vi "_Server BlockUpdate.vi"(4 "error in":errorcluster, 5 "Simulator":bool, 6 "Lens":T1[](array[typedef]), 7 "Running":bool) -> (0 "error out":errorcluster)   [LabVIEW 2015]
uses:
  Type/_XML Lens.ctl
  Type/_RT Active Ch.ctl
  Type/_RT Parameter.ctl
  Type/_RT Expt.ctl
  Type/_Run Mode.ctl
  Type/_RT Mass Range.ctl
  Type/_RT Res Type.ctl
  Type/_RT Command.ctl
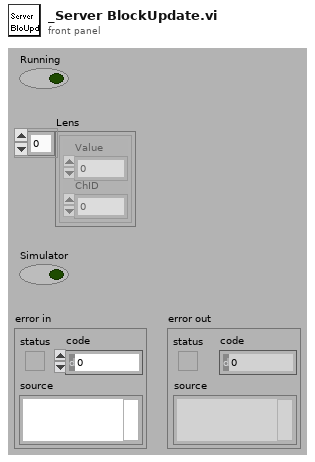
[diagram p1: front panel]
types:
  T1 = typedef "_XML Lens.ctl" = cluster{"Value":dbl, "ChID":u8}
  T2 = typedef "_RT Command.ctl" = enum16{"xml Start Run", "xml Start Actual Run", "xml Stop Run", "xml Runtime Update", "xml Get Status", "xml Get Table", "xml Set Table", "xml Get Configuration", "xml System Status", "xml Set LC Input Logic", "xml Get Data", "xml Get Info", "Start", "StartActualRun", "Stop", "Runtime Update", "Get Data", "Get Info", "Get Status", "Get Param", "Get Config", "Get Table", "Read ADC", "Set Oscillator", "Update Config", "Update Table", "Set All Pol", "Set Pol and DC", "Set Max Mass", "Toggle RP", "Toggle EL", "Set PIC", "Initialize Turbo", "Send Turbo Comm", "Close Turbo", "P1", "P2", "P3", "Send Serial", "Set LC Out", "Get LC In", "Read VAC", "Test Table", "Toggle Power", "Get Startup", "Set Startup", "Get ADC Table", "Set ADC Table", "Get Brief Status", "Get Detail Status", "Auxiliary Update", "Set CC Logics", "Set CC Input Logics", "Ignore Error", "invalid"}
  T3 = typedef "_RT Active Ch.ctl" = cluster{"Start":i32, "Step":i32, "ChID":i32}
  T4 = typedef "_RT Configuration 2.ctl" = cluster{"Name":string, "Ch#":u8, "Min":dbl, "Max":dbl, "Def+":dbl, "Def-":dbl, "Offset":dbl, "Slope":dbl, "Type":u8, "Description":string, "SettleT":dbl}
  T5 = typedef "_RT Expt.ctl" = cluster{"StartT(mS)":i32, "#Cycles":i32, "Scan Type":T6, "PauseT(uS)":i32, "Polarity":u8, "DelayT(mS)":i32, "Active Ch":T3[], "Mass Range":T7[]}
  T6 = typedef "_Run Mode.ctl" = enum16{"MRM (Q1/Q2)", "Q1 Scan", "Q1 SRM", "Q2 Scan", "Q2 SRM", "Product Scan", "Precursor Scan", "Neutral Loss", "Neutral Gain"}
  T7 = typedef "_RT Mass Range.ctl" = cluster{"Steps":i32, "Dwell(uS)":i32, "Resolution Type":T8, "Ramping Ch":T3[]}
  T8 = typedef "_RT Res Type.ctl" = u16
  T9 = typedef "_RT Parameter.ctl" = cluster{"RunMode":i32, "Initial Ch":T3[], "Sync":u8, "Expt":T5[], "EqTime(mS)":i32}
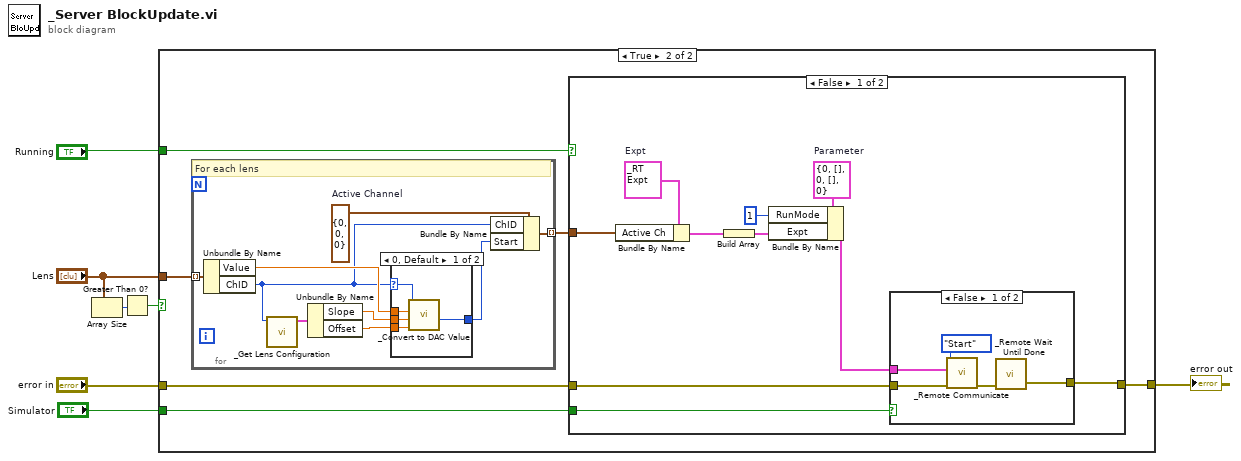
[diagram p0: block diagram]
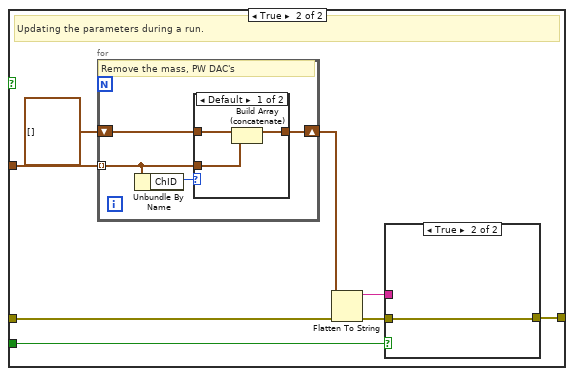
[diagram p4: hidden frame]
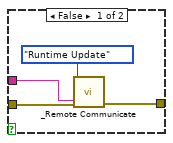
[diagram p5: hidden frame]
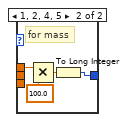
[diagram p7: hidden frame]
diagram:
  n1 = Array Size(array="Lens") -> (size(s)=w6:i32)
  n2 = Greater Than 0?(x=w6) -> (x > 0?=w5:bool)
  n3 = case shown="True" w5 {
    tunnel: "Lens" -> [_ w13]
    tunnel: "error in" -> [w8 w11]
    tunnel: [w8 w10] -> w3
    tunnel: "Running" -> [_ w12]
    tunnel: "Simulator" -> [_ w9]
    frame False {
    }
    frame True {
      n4 = for {
        tunnel: [w56] -> w14 mode=indexing
        tunnel: w13 -> [w55] mode=indexing
        w58 = T3 {"Start"=0, "Step"=0, "ChID"=0}  # Active Channel
        # "For each lens"
        n5 = Unbundle By Name(w55) -> ("Value"=w54:dbl, "ChID"=w53:u8)
        n6 = call "_Get Lens Configuration.vi"("Channel #"=w53) -> ("Lens Configuration"=w52:T4)  [unwired: 1 in, 5 out]
        n7 = Unbundle By Name(w52) -> ("Slope"=w60:dbl, "Offset"=w59:dbl)
        n8 = case shown="0, Default" w53 {
          selector: w53 -> [w61 _]
          tunnel: w54 -> [w65 w69]
          tunnel: w60 -> [w64 _]
          tunnel: w59 -> [w63 _]
          tunnel: [w62 w66] -> w57
          frame 0, Default {
            n9 = call "_Convert to DAC Value.vi"("Offset"=w63, "Slop"=w64, "Number"=w65, "Channel"=w61) -> ("DAC Value"=w62:i32)  [unwired: 2 in, 5 out]
          }
          frame 1, 2, 4, 5 {
            # "for mass"
            n10 = Multiply(x=w69, y=100.0) -> (x*y=w67:dbl)
            n11 = To Long Integer(number=w67) -> (32bit integer=w66:i32)
          }
        }
        n12 = Bundle By Name(cluster=w58, "ChID"=w53, "Start"=w57) -> (w56:T3)
      }
      n13 = case shown="False" w12 {
        tunnel: w14 -> [w18 w37]
        tunnel: w11 -> [w17 w33]
        tunnel: [w16 w34] -> w10
        tunnel: w9 -> [w15 w31]
        frame False {
          w21 = T5 {"StartT(mS)"=0, "#Cycles"=1, "Scan Type"=enum."MRM (Q1/Q2)", "PauseT(uS)"=0, "Polarity"=0, "DelayT(mS)"=0, "Active Ch"=[], "Mass Range"=[]}  # Expt
          w24 = T9 {"RunMode"=0, "Initial Ch"=[], "Sync"=0, "Expt"=[], "EqTime(mS)"=0}  # Parameter
          n14 = Bundle By Name(cluster=w21, "Active Ch"=w18) -> (w20:T5)
          n15 = Build Array(w20) -> (w19:T5[])
          n16 = Bundle By Name(cluster=w24, "RunMode"=1, "Expt"=w19) -> (w23:T9)
          n17 = case shown="False" w15 {
            tunnel: w23 -> [w27 _]
            tunnel: w17 -> [w26 w30]
            tunnel: [w25 w30] -> w16
            frame False {
              n18 = call "_Remote Communicate.vi"("error in (no error)"=w26, "Parameter"=w27, "Command"=_RT_Command."Start") -> ("error out"=w28:errorcluster)  [unwired: 3 in, 3 out]
              n19 = call "_Remote Wait Until Done.vi"("error IO"=w28) -> ("error out"=w25:errorcluster)  [unwired: 1 in, 1 out]
            }
            frame True {
            }
          }
        }
        frame True {
          # "Updating the parameters during a run."
          n20 = for {
            shift-right: [w45] -> w36
            shift-left: T3[] [] ("Array") -> [w46]
            tunnel: w37 -> [w44] mode=indexing
            # "Remove the mass, PW DAC's"
            n21 = Unbundle By Name(w44) -> ("ChID"=w47:i32)
            n22 = case shown="Default" w47 {
              tunnel: [w48 w51] -> w45
              tunnel: w46 -> [w50 w51]
              tunnel: w44 -> [w49 _]
              frame Default {
                n23 = Build Array (concatenate)(w50, w49) -> (w48:T3[])
              }
              frame 0..2, 4, 5, 7, 9 {
              }
            }
          }
          n24 = Flatten To String(anything=w36, error in (no error)=w33) -> (data string=w38:string, error out=w32:errorcluster)  [unwired: 3 out]
          n25 = case shown="True" w31 {
            tunnel: w38 -> [w41 _]
            tunnel: [w40 w43] -> w34
            tunnel: w32 -> [w39 w43]
            frame False {
              n26 = call "_Remote Communicate.vi"("String"=w41, "error in (no error)"=w39, "Command"=_RT_Command."Runtime Update") -> ("error out"=w40:errorcluster)  [unwired: 3 in, 3 out]
            }
            frame True {
            }
          }
        }
      }
    }
  }
  "error out" <- w3
